vi "Day 5.1.vi"(11 "input":string[](array[string])) -> (3 "ouptut part 1":u64)   [LabVIEW 2021]
uses:
  bd020075-89f8-4bf5-b948-f6dec5283510.vi
  <vilib>/regexp/Match Regular Expression.xnode
  <vilib>/Comparison/Less/Less Functor/Less Functor.lvclass
panel:
  out "Final locations":u64[](array[numeric])
  out "Maps":T1(array[cluster])
  out "seeds":u64[](array[numeric])
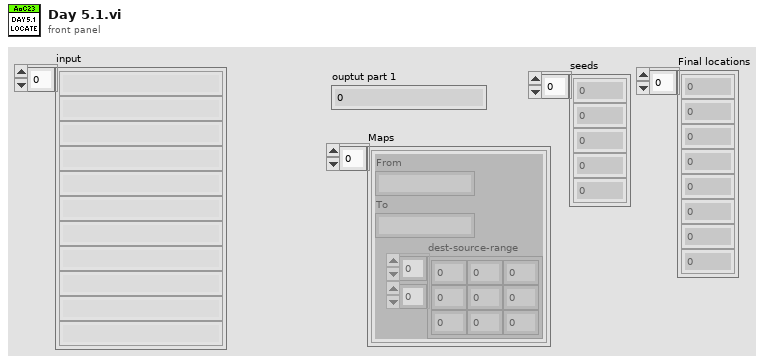
[diagram p1: front panel]
types:
  T1 = cluster{"From":string, "To":string, "dest-source-range":u64[][]}[]
  T2 = cluster{"From":string, "To":string, "dest-source-range":u64[][]}
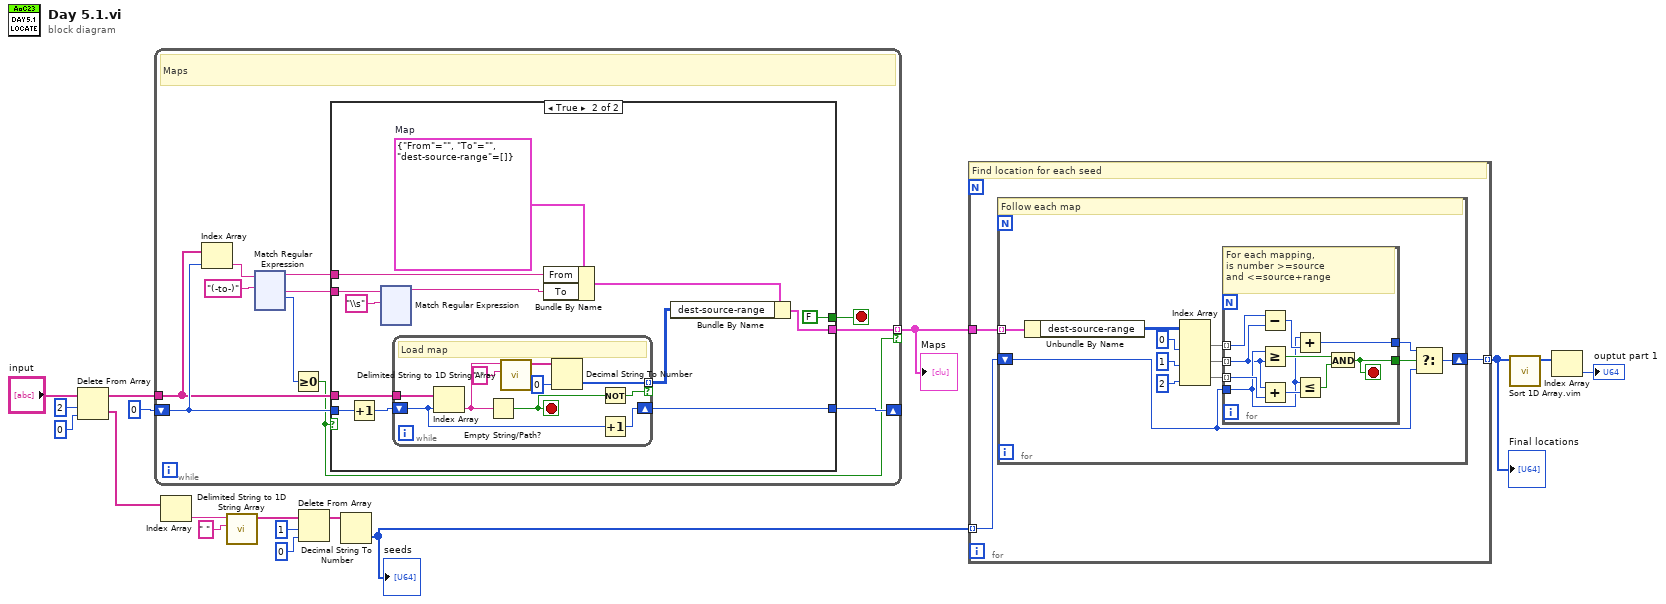
[diagram p0: block diagram]
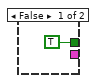
[diagram p2: hidden frame]
diagram:
  n1 = Delete From Array(array="input", length=2, index=0) -> (deleted portion=w13:string[], array with subset deleted=w15:string[])
  n2 = while {
    tunnel: w15 -> [w23]
    shift-right: [w22] -> _
    shift-left: 0 -> [w24]
    tunnel: [w21] -> w4 mode=indexing if=w19
    stop <- w18 stop-if-true
    # "Maps"
    n3 = Index Array(array=w23, index=w24) -> (element=w25:string)
    n4 = xnode "Match Regular Expression"("input string"=w25, "regular expression"="(-to-)") -> ("before match"=w27:string, "after match"=w26:string, "offset past match"=w20:i32)  [unwired: 4 in, 2 out]
    n5 = Greater Or Equal To 0?(x=w20) -> (x >= 0?=w19:bool)
    n6 = case shown="True" w19 {
      tunnel: w27 -> [_ w41]
      tunnel: w26 -> [_ w40]
      tunnel: w24 -> [_ w37]
      tunnel: w23 -> [_ w35]
      tunnel: [_ w32] -> w22
      tunnel: [_ w31] -> w21
      tunnel: [TRUE FALSE] -> w18
      frame False {
      }
      frame True {
        w42 = T2 {"From"="", "To"="", "dest-source-range"=[]}  # Map
        n7 = Increment(x=w37) -> (x+1=w36:i32)
        n8 = xnode "Match Regular Expression"("input string"=w40, "regular expression"="\\s") -> ("before match"=w38:string)  [unwired: 4 in, 4 out]
        n9 = while {
          shift-right: [w44] -> w32
          shift-left: w36 -> [w45]
          tunnel: w35 -> [w52]
          tunnel: [w48] -> w33 mode=indexing if=w46
          stop <- w47 stop-if-true
          # "Load map"
          n10 = Index Array(array=w52, index=w45) -> (element=w50:string)
          n11 = Empty String/Path?(string/path=w50) -> (empty?=w47:bool)
          n12 = call <vilib>:"Delimited String to 1D String Array.vi"("delimiter"=" ", "delimited string"=w50) -> ("string array"=w49:string[])  [unwired: 9 in]
          n13 = Decimal String To Number(string=w49, default (0L)=u64 0 ("default (0 I32)")) -> (number=w48:u64[])  [unwired: 1 in, 1 out]
          n14 = Not(x=w47) -> (.not. x?=w46:bool)
          n15 = Increment(x=w45) -> (x+1=w44:i32)
        }
        n16 = Bundle By Name(cluster=w42, "From"=w41, "To"=w38) -> (w34:T2)
        n17 = Bundle By Name(cluster=w34, "dest-source-range"=w33) -> (w31:T2)
      }
    }
  }
  "Maps" <- w4
  n18 = Index Array(array=w13) -> (element=w12:string)  [unwired: 1 in]
  n19 = call <vilib>:"Delimited String to 1D String Array.vi"("delimiter"=" ", "delimited string"=w12) -> ("string array"=w10:string[])  [unwired: 9 in]
  n20 = Delete From Array(array=w10, length=1, index=0) -> (array with subset deleted=w7:string[])  [unwired: 1 out]
  n21 = Decimal String To Number(string=w7) -> (number=w5:i32[])  [unwired: 2 in, 1 out]
  "seeds" <- w5
  n22 = for {
    tunnel: w5 -> [w288] mode=indexing
    tunnel: w4 -> [w289]
    tunnel: [w287] -> w3 mode=indexing
    # "Find location for each seed"
    n23 = for {
      tunnel: w289 -> [w301] mode=indexing
      shift-right: [w290] -> w287
      shift-left: w288 -> [w291]
      # "Follow each map"
      n24 = Unbundle By Name(w301) -> ("dest-source-range"=w300:u64[][])
      n25 = Index Array(array=w300, index (col) #1=0 ("disabled index (col)"), index (col) #2=1 ("index (col)"), index (col) #3=2 ("index (col)")) -> (element #1=w296:u64[], element #2=w295:u64[], element #3=w294:u64[])  [unwired: 3 in]
      n26 = for {
        tunnel: w296 -> [w304] mode=indexing
        tunnel: w295 -> [w302] mode=indexing
        tunnel: w294 -> [w311] mode=indexing
        tunnel: w291 -> [w303]
        tunnel: [w306] -> w292
        tunnel: [w305] -> w293
        stop <- w305 stop-if-true
        # "For each mapping,\nis number >=source\nand <=source+range"
        n27 = Subtract(x=w304, y=w302) -> (x-y=w307:u64)
        n28 = Greater Or Equal?(x=w303, y=w302) -> (x >= y?=w309:bool)
        n29 = Add(x=w302, y=w311) -> (x+y=w310:u64)
        n30 = Add(x=w303, y=w307) -> (x+y=w306:u64)
        n31 = Less Or Equal?(x=w303, y=w310) -> (x <= y?=w308:bool)
        n32 = And(x=w309, y=w308) -> (x .and. y?=w305:bool)
      }
      n33 = Select(t=w292, s=w293, f=w291) -> (s? t:f=w290:u64)
    }
  }
  "Final locations" <- w3
  n34 = call "Sort 1D Array.vim"("unsorted array"=w3) -> ("sorted array"=w2:u64[])  [unwired: 10 in]
  n35 = Index Array(array=w2) -> (element=→"ouptut part 1":u64)  [unwired: 1 in]
